vi "RequestInsertEvents.vi"(5 "Events":T1[](array[typedef]), 11 "error in (no error)":errorcluster) -> (6 "request":string, 15 "error out":errorcluster)   [LabVIEW 2019, in "Logger.lvclass"]
uses:
  Logger.lvclass
  EventData.ctl
  EventType.ctl
  TypeDef/AlarmType.ctl
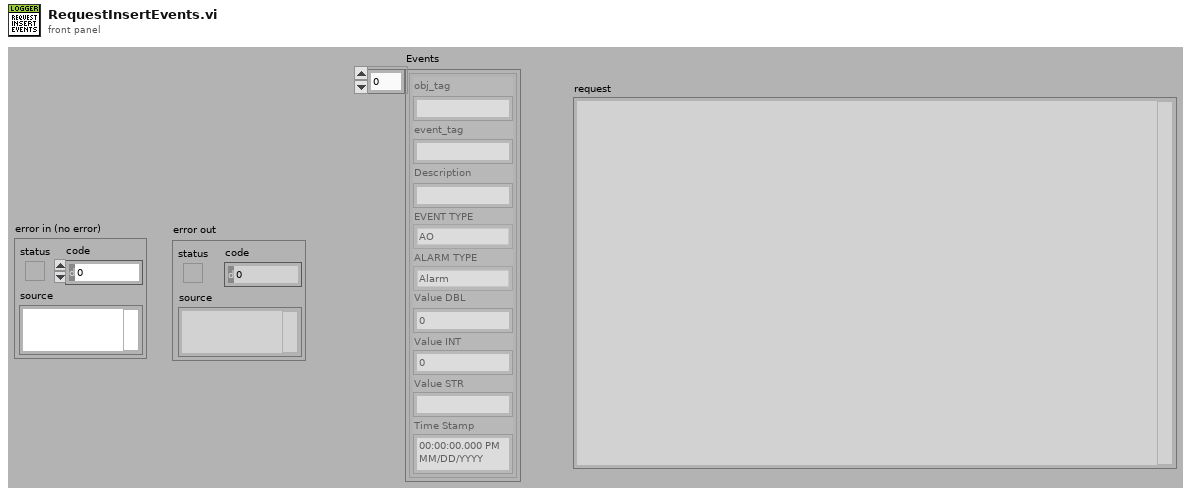
[diagram p1: front panel]
types:
  T1 = typedef "Logger.lvclass/EventData.ctl" = cluster{"obj_tag":string, "event_tag":string, "Description":string, "EVENT TYPE":T2, "ALARM TYPE":T3, "Value DBL":dbl, "Value INT":i32, "Value STR":string, "Time Stamp":timestamp}
  T2 = typedef "Logger.lvclass/EventType.ctl" = enum16{"DI", "DO", "DA", "AI", "AO", "AA", "CMD", "ERR", "ST"}
  T3 = typedef "AlarmType.ctl" = enum16{"Normal", "Warning", "Alarm"}
  T4 = typedef "Logger.lvclass/EventCode.ctl" = enum16{"DI_EU_LO", "DI_EU_HI", "DIO_LO", "DIO_HI", "DI_RAW_LO", "DI_RAW_HI", "DO_LO", "DO_HI", "DA_OK", "DA_ALARM", "AA_HI", "AA_HIHI", "AA_LO", "AA_LOLO", "AA_OK", "CMD", "OUT_OF_RANGE_OK", "OUT_OF_RANGE_LO", "OUT_OF_RANGE_HI", "CONFIG", "DI_LO", "DI_HI"}
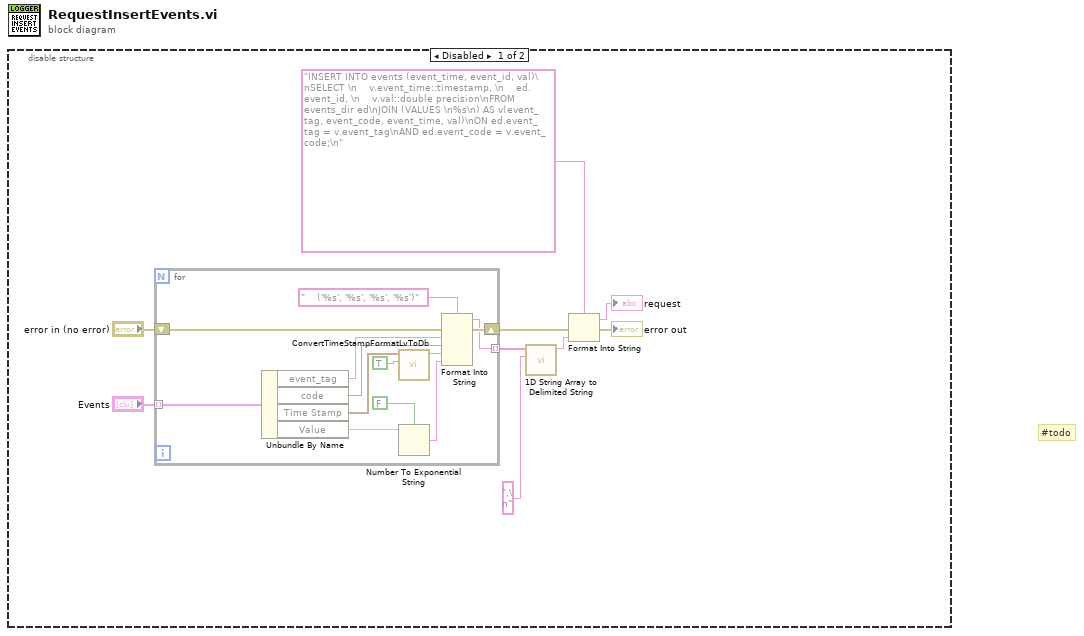
[diagram p0: block diagram]
diagram:
  # "#todo"
  n1 = disable-structure shown="Disabled" {
    frame Disabled {
      n2 = for {
        tunnel: [w21] -> w8 mode=indexing
        tunnel: "Events" -> [w18] mode=indexing
        shift-right: [w22] -> w3
        shift-left: "error in (no error)" -> [w20]
        n3 = Unbundle By Name(w18) -> ("event_tag"=w17:string, "code"=w16:T4, "Time Stamp"=w15:timestamp, "Value"=w12:dbl)
        n4 = call "ConvertTimeStampFormatLvToDb.vi"("to UTC (F)"=TRUE, "Time Stamp"=w15) -> ("output string"=w14:string)  [unwired: 9 in]
        n5 = Number To Exponential String(number=w12, 1:FALSE ("use system decimal point (T)")) -> (E-format string=w11:string)  [unwired: 2 in]
        n6 = Format Into String(format string="    ('%s', '%s', '%s', '%s')", error in=w20, w17, w16, w14, w11) -> (resulting string=w21:string, error out=w22:errorcluster)  [unwired: 1 in]
      }
      n7 = call <vilib>:"1D String Array to Delimited String.vi"("delimiter"=",\n", "string array"=w8) -> ("delimited string"=w4:string)  [unwired: 9 in]
      n8 = Format Into String(format string="INSERT INTO events (event_time, event_id, val)\nSELECT \n    v.event_time::timestamp, \n    ed.event_id, \n    v.val::double precision\nFROM events_dir ed\nJOIN (VALUES \n%s\n) AS v(event_tag, event_code, event_time, val)\nON ed.event_tag = v.event_tag\nAND ed.event_code = v.event_code;\n", error in=w3, w4) -> (resulting string=→"request":string, error out=→"error out":errorcluster)  [unwired: 1 in]
    }
    frame Enabled {
    }
  }
